vi "Auto Shift.vi"(9 "Throttle":dbl, 11 "Manual Low Gear":bool) -> (3 "High Gear":bool)   [LabVIEW 2015]
uses:
  Common Code/Auto Shift State.ctl
  Robot Global Data.vi
panel:
  out "Throttle Accel":dbl
  out "Accel":dbl
  out "State":T1=enum."High"
  out "Speed":dbl
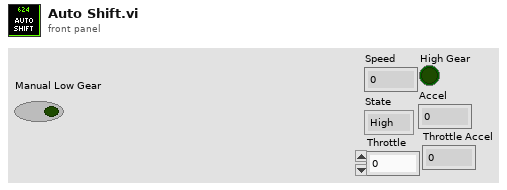
[diagram p1: front panel]
types:
  T1 = typedef "Auto Shift State.ctl" = enum16{"Low", "High"}
  T2 = typedef "Dashboard Control Data.ctl" = cluster{"Shooter Presets":T3, "Encoder Control":T5, "Steer PID output":cluster{"output high":dbl, "output low":dbl}, " Steer PID gains":cluster{"proportional gain (Kc)":dbl, "integral time (Ti, min)":dbl, "derivative time (Td, min)":dbl}, "Drivetrain Settings":T6, "Vision Packet":T7, "Dashboard Drivetrain Command":T8, "Info/Command Cluster":T10, "Ball Vision Packet":T11, "Intake Presets":T13, "Intake Encoder Control":T15, "Climb Presets":T16, "Goal Output Range":cluster{"output high":dbl, "output low":dbl}, "Enabled Systems":T17, "Auton Presets":T18, "Pressure M":dbl, "Pressure B":dbl, "Vision Timeout":dbl, "Auto-Shift":T19}
  T3 = typedef "Shooter Presets.ctl" = cluster{"Batter Shot":T4, "Deep Middle":T4, "Manual Shot":T4, "Left Ticks Per Rotation":dbl, "Right Ticks Per Rotation":dbl, "Low Bar Shot":T4, "Shooter RPM Tolerance":dbl, "Trigger Power":dbl, "Fire from Load Delay":i32, "Max Angle":dbl, "Min Angle":dbl, "Angle PID gains":cluster{"P":dbl, "I":dbl, "D":dbl}, "Angle Output":cluster{"output high":dbl, "output low":dbl}, "Shooter Angle Tolerance":dbl, "Vision Shoot x^2":dbl, "Vision Shoot x":dbl, "Feed Forward Max Accel":dbl, "Feed Forward Kv":dbl, "Backwards Trigger":dbl, "Shot Finish Delay (ms)":dbl, "Angle Max Current":dbl, "Angle Current Trip Time":dbl, "Intake Angle":dbl, "Vision Shoot c":dbl, "Reset?":bool, "Button Release Delay":dbl, "Angle Pot x":dbl, "Angle Pot c":dbl, "Ignore Angle?":bool, "Max RPM":dbl, "Safty Frist Angle":dbl, "Intake Danger Height":dbl, "Angle Pot B":i32, "Angle Pot M":dbl, "FF Finish RPM":dbl, "RPM PID Right":cluster{"P":dbl, "I":dbl, "D":dbl, "FF":dbl}, "RPM PID Left":cluster{"P":dbl, "I":dbl, "D":dbl, "FF":dbl}, "Backwards RPM":dbl, "Vision RPM":dbl, "Run Wheels Backward Delay":u32, "Cleat Shot":T4}
  T4 = typedef "Shot Presets.ctl" = cluster{"L":dbl, "R":dbl, "A":dbl}
  T5 = typedef "Encoder Control.ctl" = cluster{"Right Tick Constant":dbl, "Left Tick Constant":dbl, "Reset?":bool, "Y Dist":cluster{"PID gains":cluster{"proportional gain (Kc)":dbl, "integral time (Ti, min)":dbl, "derivative time (Td, min)":dbl}}, "Y Stop Thresh":dbl, "Y Stop Speed":dbl}
  T6 = typedef "Drivetrain Settings.ctl" = cluster{"Gyro Tolerance":dbl, "Throttle Ramp (ms)":dbl, "Kv":dbl, "Ka":dbl, "Feed Forward P":dbl, "Feed Forward D":dbl, "Goal Vision PID gains":cluster{"proportional gain (Kc)":dbl, "integral time (Ti, min)":dbl, "derivative time (Td, min)":dbl}, "Goal Detection Window":dbl, "Creep Rate":dbl, "Vision Throttle Threshold":dbl, "Min Turn Output":dbl, "Left Batter Angle":dbl, "Right Batter Angle":dbl}
  T7 = typedef "Goal Vision Packet.ctl" = cluster{"Distance":dbl, "Center X":dbl, "Center Y":dbl, "Found Target?":bool, "Robot Center":dbl, "Angle":dbl}
  T8 = typedef "Dashboard Drivetrain Command.ctl" = cluster{"Drivetrain Vision":T9}
  T9 = typedef "Drivetrain Vision.ctl" = cluster{"Goal Window":dbl, "Ball Window":dbl}
  T10 = typedef "Ball Tracking Command Cluster.ctl" = cluster{"Distance to Ball":dbl, "Desired Angle":dbl, "Command":enum16{"Turn to Ball", "Turn to Angle", "Get Distance"}, "Pixels from Center":dbl}
  T11 = typedef "Ball Vision Packet.ctl" = cluster{"Ball Detected?":bool, "Distance to Ball":dbl, "Desired Angle":dbl, "Pixels from Center":dbl, "Tracking mode":T12}
  T12 = typedef "Tracking Mode.ctl" = enum16{"Turn to Ball", "Turn to Angle"}
  T13 = typedef "Intake Presets.ctl" = cluster{"Intake Speed":dbl, "Outake Speed":dbl, "Low Height":dbl, "Half Height":dbl, "High Idle Height":dbl, "Angle Speed":dbl, "Angle Tolerance":dbl, "Encoder Scale":dbl, "Load Height":dbl, "Output Range":T14, "Rotation Power Max/Min":dbl, "MaxCurrent":dbl, "Intake Trip Time":dbl, "Idle Height":dbl, "Max Height":dbl, "Reset Encoders?":bool, "PID gains":cluster{"proportional gain (Kc)":dbl, "integral time (Ti, min)":dbl, "derivative time (Td, min)":dbl}, "Intake Stop Delay":u32, "Settle Time":dbl, "Settle Wait Time":dbl, "Pull Up Delay":dbl}
  T14 = typedef "Drivetrain Output Range.ctl" = cluster{"output high":dbl, "output low":dbl}
  T15 = typedef "IntakeEcoderControl.ctl" = cluster{"Arm Tick Constant":dbl, "Reset?":bool, "Y Dist":cluster{"PID gains":cluster{"proportional gain (Kc)":dbl, "integral time (Ti, min)":dbl, "derivative time (Td, min)":dbl}}, "Y Stop Thresh":dbl, "Y Stop Speed":dbl}
  T16 = typedef "Climb Presets.ctl" = cluster{"Pull Power":dbl, "Extend Power":dbl}
  T17 = typedef "Enabled Systems.ctl" = cluster{"Shoot":bool, "Intake":bool, "DT":bool, "Gyro":bool, "100ms":bool, "US":bool}
  T18 = typedef "Autonomous Presets.ctl" = cluster{"Pitch Limit":dbl, "Roll Limit":dbl, "Start Position":dbl, "Cross Position":dbl}
  T19 = typedef "Auto Shift Cluster.ctl" = cluster{"Delay":dbl, "Speed Thresh":dbl, "Upshift Accel":dbl, "Upshift Throttle":dbl, "Upshift Throttle Accel":dbl, "Downshift Throttle":dbl, "Downshift Throttle Accel":dbl}
  T20 = typedef "Encoder Values Super Cluster.ctl" = cluster{"Left Encoder":T21, "Right Encoder":T21}
  T21 = typedef "Encoder Values.ctl" = cluster{"Distance":dbl, "Speed":dbl, "Ticks":dbl}
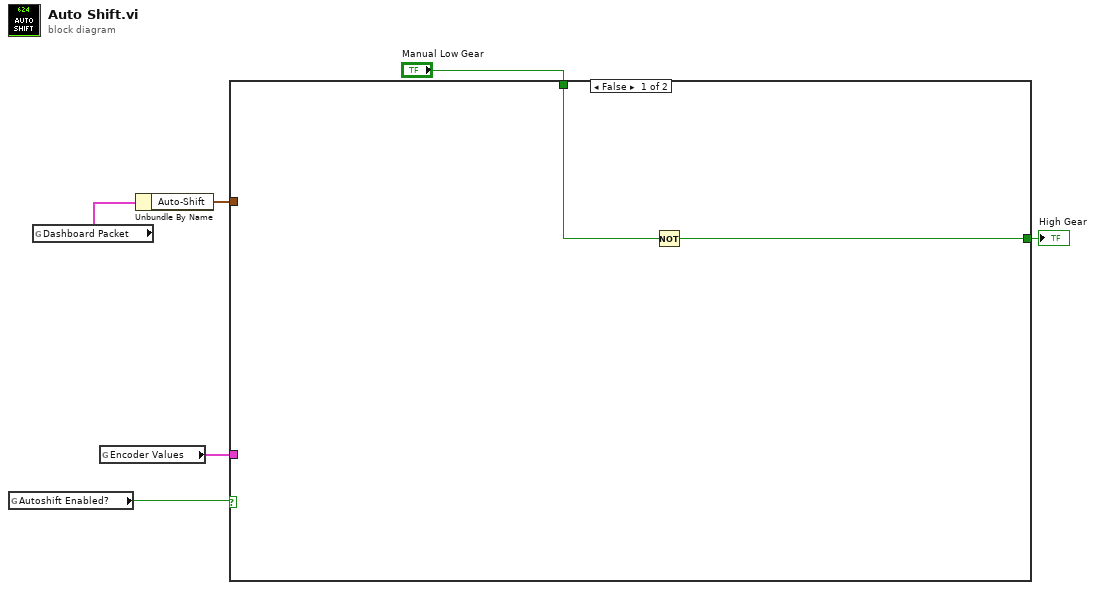
[diagram p0: block diagram]
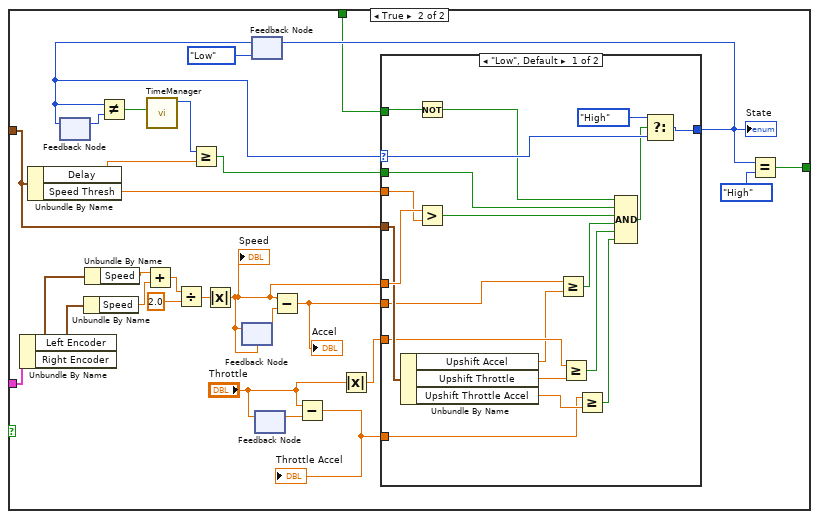
[diagram p2: hidden frame]
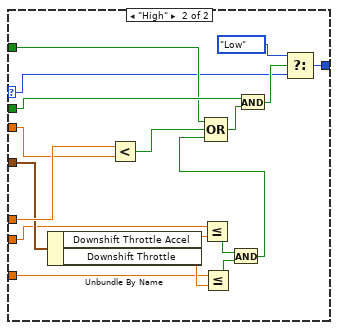
[diagram p3: hidden frame]
diagram:
  n1 = global read "Robot Global Data.vi" "Autoshift Enabled?"() -> (w1:bool)
  n2 = global read "Robot Global Data.vi" "Dashboard Packet"() -> (w6:T2)
  n3 = global read "Robot Global Data.vi" "Encoder Values"() -> (w4:T20)
  n4 = Unbundle By Name(w6) -> ("Auto-Shift"=w5:T19)
  n5 = case shown="False" w1 {
    tunnel: w5 -> [_ w13]
    tunnel: w4 -> [_ w36]
    tunnel: [w7 w19] -> w3
    tunnel: "Manual Low Gear" -> [w8 w14]
    frame False {
      n6 = Not(x=w8) -> (.not. x?=w7:bool)
    }
    frame True {
      n7 = Unbundle By Name(w36) -> ("Left Encoder"=w35:T21, "Right Encoder"=w34:T21)
      n8 = Unbundle By Name(w13) -> ("Delay"=w23:dbl, "Speed Thresh"=w17:dbl)
      n9 = feedback #1() -> (w26:T1)  [unwired: 1 in]
      n10 = Unbundle By Name(w34) -> ("Speed"=w32:dbl)
      n11 = Unbundle By Name(w35) -> ("Speed"=w33:dbl)
      n12 = Add(x=w33, y=w32) -> (x+y=w31:dbl)
      n13 = Divide(x=w31, y=2.0) -> (x/y=w29:dbl)
      n14 = Absolute Value(x=w29) -> (abs(x)=w16:dbl)
      "Speed" <- w16
      n15 = feedback-in #2(w16) -> ()
      n16 = feedback #2(w16) -> (w28:dbl)
      n17 = feedback #3(Auto_Shift_State."Low") -> (w22:T1)
      n18 = feedback-in #1(w22) -> ()
      n19 = Not Equal?(x=w22, y=w26) -> (x != y?=w25:bool)
      n20 = call "TimeManager.vi"("Reset?"=w25) -> ("Time Since Reset"=w24:u32)  [unwired: 9 in, 1 out]
      n21 = Greater Or Equal?(x=w24, y=w23) -> (x >= y?=w21:bool)
      n22 = feedback #4() -> (w12:dbl)  [unwired: 1 in]
      n23 = feedback-in #4("Throttle") -> ()
      n24 = Subtract(x=w16, y=w28) -> (x-y=w15:dbl)
      "Accel" <- w15
      n25 = Subtract(x="Throttle", y=w12) -> (x-y=w9:dbl)
      "Throttle Accel" <- w9
      n26 = Absolute Value(x="Throttle") -> (abs(x)=w10:dbl)
      n27 = case shown="\"Low\", Default" w22 {
        selector: w22 -> [w56 w70]
        tunnel: w21 -> [w51 w72]
        tunnel: [w55 w68] -> w18
        tunnel: w17 -> [w53 w65]
        tunnel: w16 -> [w54 w66]
        tunnel: w15 -> [w40 w60]
        tunnel: w14 -> [w48 w71]
        tunnel: w13 -> [w46 w64]
        tunnel: w10 -> [w42 w62]
        tunnel: w9 -> [w43 _]
        frame "Low", Default {
          n28 = Unbundle By Name(w46) -> ("Upshift Accel"=w41:dbl, "Upshift Throttle"=w45:dbl, "Upshift Throttle Accel"=w44:dbl)
          n29 = Not(x=w48) -> (.not. x?=w47:bool)
          n30 = Greater?(x=w54, y=w53) -> (0:w52:bool)
          n31 = Greater Or Equal?(x=w40, y=w41) -> (x >= y?=w39:bool)
          n32 = Greater Or Equal?(x=w42, y=w45) -> (x >= y?=w38:bool)
          n33 = Greater Or Equal?(x=w43, y=w44) -> (x >= y?=w37:bool)
          n34 = Compound Arithmetic op=AND(w47, w51, w52, w39, w38, w37) -> (w50:bool)
          n35 = Select(t=Auto_Shift_State."High", s=w50, f=w56) -> (s? t:f=w55:T1)
        }
        frame "High" {
          n36 = Unbundle By Name(w64) -> ("Downshift Throttle Accel"=w61:dbl, "Downshift Throttle"=w63:dbl)
          n37 = Less?(x=w66, y=w65) -> (x < y?=w67:bool)
          n38 = Less Or Equal?(x=w60, y=w61) -> (x <= y?=w59:bool)
          n39 = Less Or Equal?(x=w62, y=w63) -> (x <= y?=w58:bool)
          n40 = And(x=w59, y=w58) -> (x .and. y?=w57:bool)
          n41 = Compound Arithmetic op=OR(w71, w67, w57) -> (w74:bool)
          n42 = And(x=w72, y=w74) -> (x .and. y?=w73:bool)
          n43 = Select(t=Auto_Shift_State."Low", s=w73, f=w70) -> (s? t:f=w68:T1)
        }
      }
      "State" <- w18
      n44 = feedback-in #3(w18) -> ()
      n45 = Equal?(x=w18, y=Auto_Shift_State."High") -> (x = y?=w19:bool)
    }
  }
  "High Gear" <- w3
